vi "Teszt cluster2string.vi"(11 "Teszt cluster":T1) -> (2 "Etalon string array":string[](array[string]), 3 "Teszt vektor string array":string[](array[string]))   [LabVIEW 2014]
uses:
  Teszt.ctl
  Command.ctl
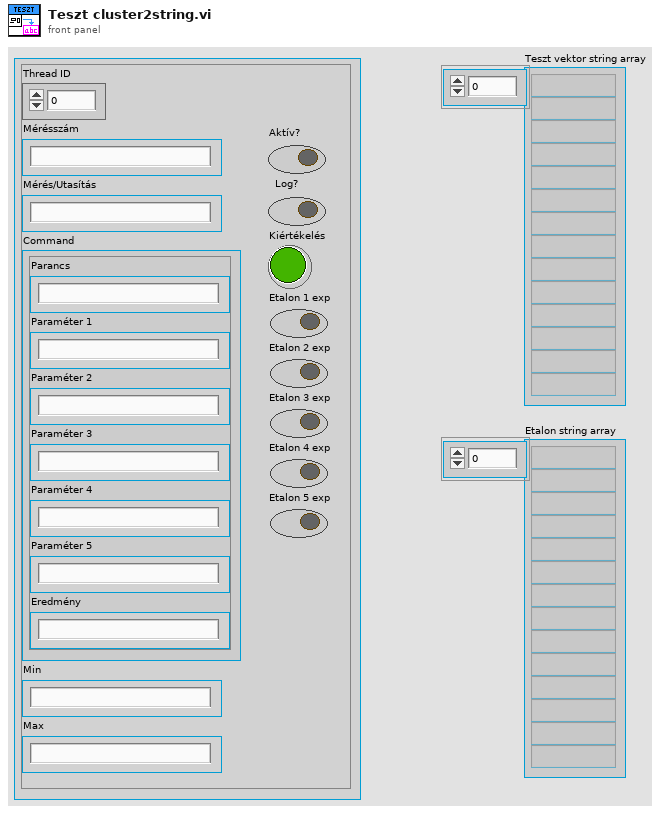
[diagram p1: front panel]
types:
  T1 = typedef "Teszt.ctl" = cluster{"Thread ID":dbl, "Mérésszám":string, "Mérés/Utasítás":string, "Command":T2, "Min":string, "Max":string, "Aktív?":bool, "Log?":bool, "Kiértékelés":bool, "Etalon 1 exp":bool, "Etalon 2 exp":bool, "Etalon 3 exp":bool, "Etalon 4 exp":bool, "Etalon 5 exp":bool}
  T2 = typedef "Command.ctl" = cluster{"Parancs":string, "Paraméter 1":string, "Paraméter 2":string, "Paraméter 3":string, "Paraméter 4":string, "Paraméter 5":string, "Eredmény":string}
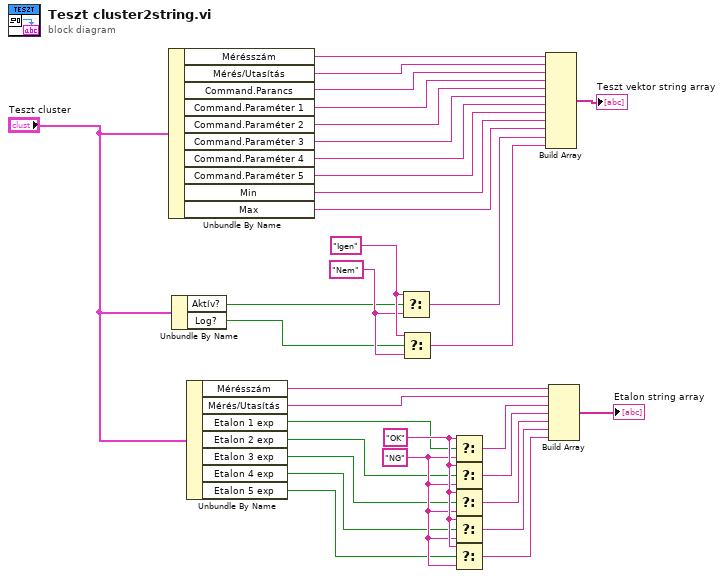
[diagram p0: block diagram]
diagram:
  w11 = "NG"
  w12 = "OK"
  w29 = "Nem"
  w30 = "Igen"
  n1 = Unbundle By Name("Teszt cluster") -> ("Mérésszám"=w31:string, "Mérés/Utasítás"=w33:string, "Command.Parancs"=w26:string, "Command.Paraméter 1"=w25:string, "Command.Paraméter 2"=w24:string, "Command.Paraméter 3"=w23:string, "Command.Paraméter 4"=w22:string, "Command.Paraméter 5"=w21:string, "Min"=w20:string, "Max"=w17:string)
  n2 = Unbundle By Name("Teszt cluster") -> ("Aktív?"=w28:bool, "Log?"=w27:bool)
  n3 = Unbundle By Name("Teszt cluster") -> ("Mérésszám"=w14:string, "Mérés/Utasítás"=w13:string, "Etalon 1 exp"=w10:bool, "Etalon 2 exp"=w9:bool, "Etalon 3 exp"=w8:bool, "Etalon 4 exp"=w7:bool, "Etalon 5 exp"=w6:bool)
  n4 = Select(t=w30, s=w28, f=w29) -> (s? t:f=w19:string)
  n5 = Select(t=w30, s=w27, f=w29) -> (s? t:f=w18:string)
  n6 = Select(t=w12, s=w10, f=w11) -> (s? t:f=w5:string)
  n7 = Select(t=w12, s=w9, f=w11) -> (s? t:f=w4:string)
  n8 = Select(t=w12, s=w8, f=w11) -> (s? t:f=w3:string)
  n9 = Select(t=w12, s=w7, f=w11) -> (s? t:f=w2:string)
  n10 = Select(t=w12, s=w6, f=w11) -> (s? t:f=w1:string)
  n11 = Build Array(w31, w33, w26, w25, w24, w23, w22, w21, w20, w17, w19, w18) -> (→"Teszt vektor string array":string[])
  n12 = Build Array(w14, w13, w5, w4, w3, w2, w1) -> (→"Etalon string array":string[])
